vi "core_timing_example_FGV.vi"(2 "data":dbl=nan format="%#_13g") -> (7 "data":dbl)   [LabVIEW 2015]
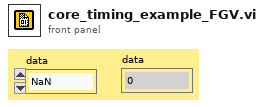
[diagram p1: front panel]
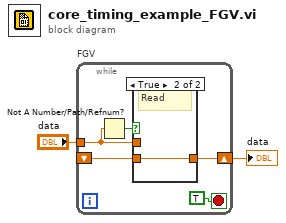
[diagram p0: block diagram]
diagram:
  n1 = while "FGV" {
    tunnel: "data" -> [w4]
    shift-right: [w6] -> w1
    shift-left: _ -> [w5]
    stop <- TRUE stop-if-true
    n2 = Not A Number/Path/Refnum?(number/path/refnum=w4) -> (NaN/Path/Refnum?=w3:bool)
    n3 = case shown="True" w3 {
      tunnel: w4 -> [w8 _]
      tunnel: [w8 w9] -> w6
      tunnel: w5 -> [_ w9]
      frame False {
        # "Write"
      }
      frame True {
        # "Read"
      }
    }
  }
  "data" <- w1
